vi "Destroy.vi"(0 "reference in":refnum<class "HeatingSystem.lvclass">, 5 "Error In":errorcluster) -> (14 "reference out":refnum<class "HeatingSystem.lvclass">, 19 "Error Out":errorcluster)   [LabVIEW 2024, in "HeatingSystem.lvclass"]
uses:
  HeatingSystem.lvclass/HeatingSystem.ctl
  HeatingSystem.lvclass
panel:
  # "Connector Pane"
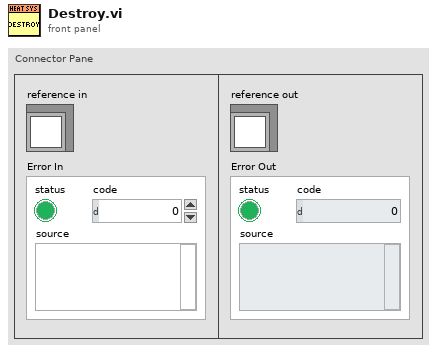
[diagram p1: front panel]
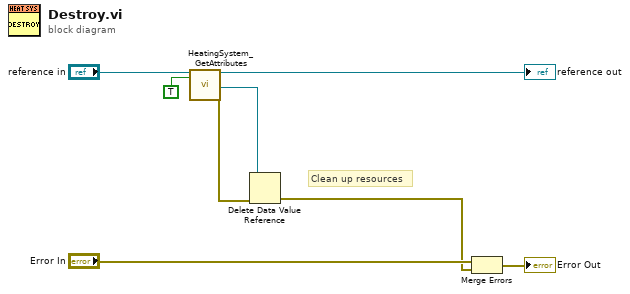
[diagram p0: block diagram]
diagram:
  # "Clean up resources"
  n1 = call "HeatingSystem_GetAttributes.vi"("reference in"="reference in", "OnlyGetDvrReference(False)"=TRUE) -> ("reference out"=→"reference out":refnum<class "HeatingSystem.lvclass">, "DataRef"=w4:refnum<data-value>, "Error Out"=w5:errorcluster)  [unwired: 14 in, 1 out]
  n2 = Delete Data Value Reference(data value reference=w4, error in=w5) -> (error out=w2:errorcluster)  [unwired: 1 out]
  n3 = Merge Errors("Error In", w2) -> (→"Error Out":errorcluster)
